vi "LoopAndQueryOutput.vi"(0 "VISA Refnum in":refnum<visa-resource-name>, 1 "Output channel selection":T1, 2 "error in (no error)":errorcluster) -> (3 "VISA resource name out":refnum<visa-resource-name>, 4 "Setpoint / V":dbl[](array[numeric]), 5 "Control signal / V":dbl[](array[numeric]), 6 "error out":errorcluster)   [LabVIEW 2015]
doc: "Loop through a selection of output channels and query the device for each one that is selected"
uses:
  controls/ChannelSelection.ctl
  Driver/Typedefs/OutputChannelTypedef.ctl
  Driver/YbTempCtrl.lvlib
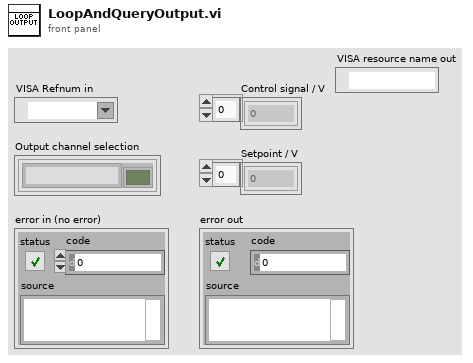
[diagram p1: front panel]
types:
  T1 = typedef "ChannelSelection.ctl" = cluster{"Channel name":string, "Enum id":u16, "Logging?":bool}[]
  T2 = typedef "YbTempCtrl.lvlib/OutputChannelTypedef.ctl" = enum16{"1", "2", "3", "4", "BPA", "BPB"}
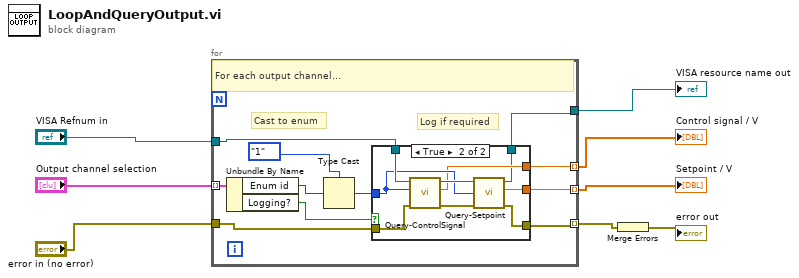
[diagram p0: block diagram]
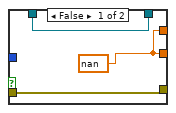
[diagram p2: hidden frame]
diagram:
  n1 = for {
    tunnel: "Output channel selection" -> [w19] mode=indexing
    tunnel: "VISA Refnum in" -> [w15]
    tunnel: [w11] -> w7 mode=indexing
    tunnel: [w10] -> w8 mode=indexing
    tunnel: [w9] -> w3
    tunnel: "error in (no error)" -> [w13]
    tunnel: [w14] -> w1 mode=indexing
    # "Log if required"
    # "Cast to enum"
    # "For each output channel..."
    n2 = Unbundle By Name(w19) -> ("Enum id"=w18:u16, "Logging?"=w17:bool)
    n3 = Type Cast(type=OutputChannelTypedef."1" ("Output channel"), x=w18) -> (*(type *) &x=w16:T2)
    n4 = case shown="True" w17 {
      tunnel: w16 -> [_ w29]
      tunnel: w15 -> [w20 w30]
      tunnel: w13 -> [w22 w28]
      tunnel: [w22 w26] -> w14
      tunnel: [w21 w25] -> w11
      tunnel: [w21 w24] -> w10
      tunnel: [w20 w23] -> w9
      frame False {
        w21 = nan ("Error Signal / V")
      }
      frame True {
        n5 = call "Query-ControlSignal.vi"("error in (no error)"=w28, "Output channel"=w29, "VISA resource name"=w30) -> ("error out"=w27:errorcluster, "Recalled Control signal / V"=w25:dbl, "VISA resource name out"=w31:refnum<visa-resource-name>)  [unwired: 6 in]
        n6 = call "Query-Setpoint.vi"("error in (no error)"=w27, "Output channel"=w29, "VISA resource name"=w31) -> ("error out"=w26:errorcluster, "Recalled setpoint / V"=w24:dbl, "VISA resource name out"=w23:refnum<visa-resource-name>)  [unwired: 3 in]
      }
    }
  }
  "Setpoint / V" <- w8
  "Control signal / V" <- w7
  "VISA resource name out" <- w3
  n7 = Merge Errors(w1) -> (→"error out":errorcluster)
